vi "create file ref for XsYa.vi"(0 "parent data folder":path, 1 "Book number":i32, 11 "error in":errorcluster) -> (4 "xml path":path, 6 "field dat":path, 8 "para dat":path, 10 "data dat":path, 15 "error out":errorcluster)   [LabVIEW 2023]
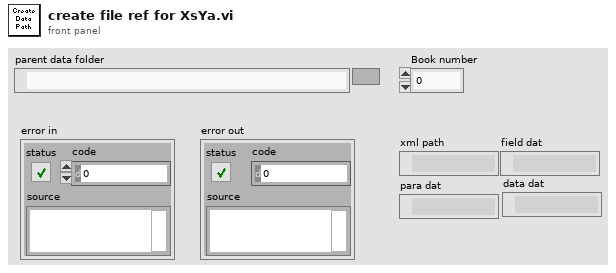
[diagram p1: front panel]
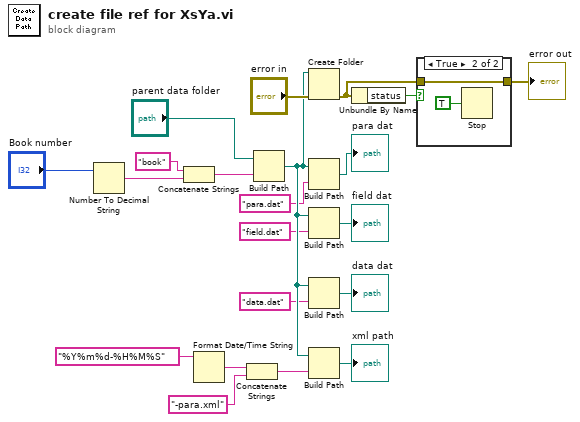
[diagram p0: block diagram]
diagram:
  n1 = Number To Decimal String(number="Book number") -> (decimal integer string=w14:string)  [unwired: 1 in]
  n2 = Concatenate Strings("book" ("string"), w14) -> (w13:string)
  n3 = Format Date/Time String(time format string (%c)="%Y%m%d-%H%M%S") -> (date/time string=w12:string)  [unwired: 2 in]
  n4 = Concatenate Strings(w12, "-para.xml" ("string")) -> (w10:string)
  n5 = Build Path(base path="parent data folder", name or relative path=w13) -> (appended path=w8:path)
  n6 = Create Folder(path (use dialog)=w8, error in="error in") -> (error out=w18:errorcluster)  [unwired: 1 in, 2 out]
  n7 = Build Path(base path=w8, name or relative path="para.dat") -> (appended path=→"para dat":path)
  n8 = Build Path(base path=w8, name or relative path="field.dat") -> (appended path=→"field dat":path)
  n9 = Build Path(base path=w8, name or relative path="data.dat") -> (appended path=→"data dat":path)
  n10 = Build Path(base path=w8, name or relative path=w10) -> (appended path=→"xml path":path)
  n11 = Unbundle By Name(w18) -> ("status"=w19:bool)
  n12 = case shown="True" w19 {
    tunnel: [w22 w24] -> w1
    tunnel: w18 -> [w22 w24]
    frame False {
    }
    frame True {
      n13 = Stop(stop? (T)=TRUE) -> ()
    }
  }
  "error out" <- w1
